vi "Periodic Tasks.vi"(8 "error in":errorcluster) -> ()   [LabVIEW 2017]
doc: "This VI runs in parallel to other tasks. It can contain as many user-defined periodic loops as you need. These can carry out PID or other sorts of timed response."
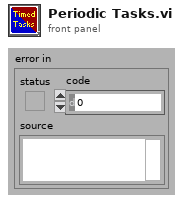
[diagram p1: front panel]
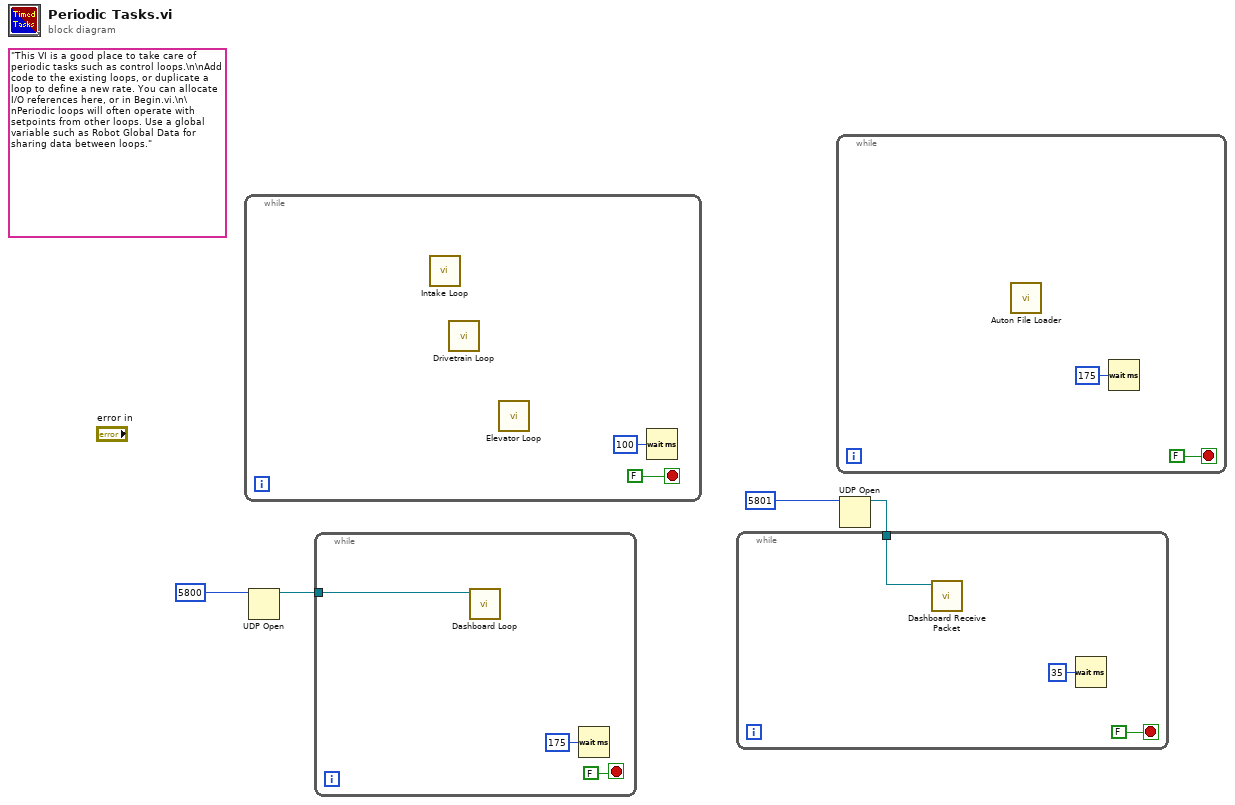
[diagram p0: block diagram]
diagram:
  (unwired) "This VI is a good place to take care of periodic tasks such as control loops.\n\nAdd code to the existing loops, or duplicate a loop to define a new rate. You can allocate I/O references here, or in Begin.vi.\n\nPeriodic loops will often operate with setpoints from other loops. Use a global variable such as Robot Global Data for sharing data between loops."
  n1 = while {
    stop <- FALSE stop-if-true
    n2 = call "Intake Loop.vi"() -> ()  [unwired: 12 in]
    n3 = call "Drivetrain Loop.vi"() -> ()  [unwired: 12 in]
    n4 = call "Elevator Loop.vi"() -> ()  [unwired: 12 in]
    n5 = Wait (ms)(milliseconds to wait=u32 100) -> ()  [unwired: 1 out]
  }
  n6 = UDP Open(11:5800) -> (port=w3:refnum<k16>)  [unwired: 4 in, 2 out]
  n7 = while {
    tunnel: w3 -> [w7]
    stop <- FALSE stop-if-true
    n8 = call "Dashboard Loop.vi"("connection ID"=w7) -> ()  [unwired: 11 in]
    n9 = Wait (ms)(milliseconds to wait=u32 175) -> ()  [unwired: 1 out]
  }
  n10 = while {
    stop <- FALSE stop-if-true
    n11 = call "Auton File Loader.vi"() -> ()  [unwired: 12 in]
    n12 = Wait (ms)(milliseconds to wait=u32 175) -> ()  [unwired: 1 out]
  }
  n13 = UDP Open(11:5801) -> (port=w1:refnum<k16>)  [unwired: 4 in, 2 out]
  n14 = while {
    tunnel: w1 -> [w14]
    stop <- FALSE stop-if-true
    n15 = call "Dashboard Receive Packet.vi"("connection ID"=w14) -> ()  [unwired: 11 in]
    n16 = Wait (ms)(milliseconds to wait=u32 35) -> ()  [unwired: 1 out]
  }
